vi "String Index Of Test Serial Output.vi"() -> ()   [LabVIEW 2014, in "ESP8266 WiFi Wrapper.lvlib"]
uses:
  <vilib>/Aledyne-TSXperts/Arduino Compatible Compiler for LabVIEW/addons/ESP8266 WiFi Wrapper/ESP8266 WiFi Wrapper.lvlib
  <vilib>/Aledyne-TSXperts/Arduino Compatible Compiler for LabVIEW/Arduino Compatible Compiler for LabVIEW.lvlib
panel:
  out "index":i8
  out "Error Out":errorcluster
  in  "Error In":errorcluster
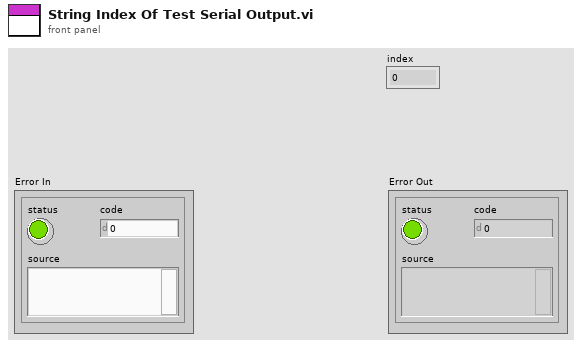
[diagram p1: front panel]
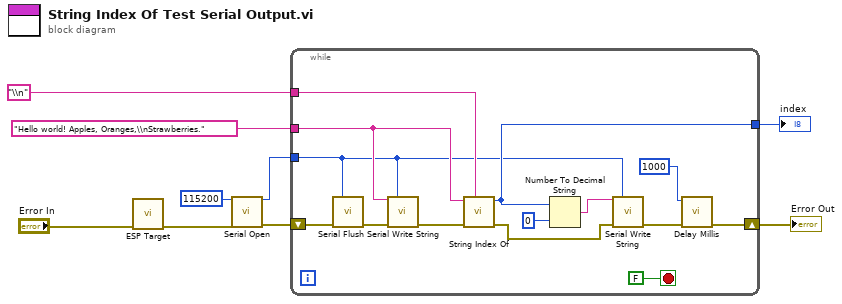
[diagram p0: block diagram]
diagram:
  n1 = call <vilib>:"ESP Target.vi"("Error In"="Error In") -> ("Error Out"=w2:errorcluster)  [unwired: 10 in]
  n2 = call <vilib>:"Serial Open.vi"("Speed"=u32 115200, "error in (no error)"=w2) -> ("Instance"=w3:u8, "error out"=w8:errorcluster)  [unwired: 12 in]
  n3 = while {
    tunnel: "\\n" ("IndexOf String") -> [w23]
    tunnel: "Hello world! Apples, Oranges,\\nStrawberries." ("Input String") -> [w20]
    tunnel: [w18] -> w4
    tunnel: w3 -> [w15]
    shift-right: [w12] -> w5
    shift-left: w8 -> [w22]
    stop <- FALSE stop-if-true
    n4 = call <vilib>:"Serial Flush.vi"("Instance"=w15, "error in (no error)"=w22) -> ("error out"=w21:errorcluster)  [unwired: 13 in]
    n5 = call <vilib>:"Serial Write String.vi"("String"=w20, "Instance"=w15, "error in (no error)"=w21) -> ("error out"=w19:errorcluster)  [unwired: 12 in]
    n6 = call <vilib>:"String Index Of.vi"("IndexOf String"=w23, "Error In"=w19, "Input String"=w20) -> ("Error Out"=w16:errorcluster, "index"=w18:i8)  [unwired: 7 in]
    n7 = Number To Decimal String(number=w18, width (-)=i16 0) -> (decimal integer string=w17:string)
    n8 = call <vilib>:"Serial Write String.vi"("String"=w17, "Instance"=w15, "error in (no error)"=w16) -> ("error out"=w13:errorcluster)  [unwired: 12 in]
    n9 = call <vilib>:"Delay Millis.vi"("error in (no error)"=w13, "delay"=u32 1000) -> ("error out"=w12:errorcluster)  [unwired: 9 in]
  }
  "Error Out" <- w5
  "index" <- w4
